vi "GetRemoteVIRef.vi"(8 "ErrorIn":errorcluster, 11 "YActorIn":refnum<class "YActor.lvclass">) -> (0 "ErrorOut":errorcluster, 1 "CreatedVI":refnum<vi>, 3 "YActorOut":refnum<class "YActor.lvclass">)   [LabVIEW 2021, in "YActor.lvclass"]
uses:
  YActor.lvclass
  YActor.lvclass/YActor.ctl
  InlineReferencePool.ctl
  ExeCmd_sync.vi
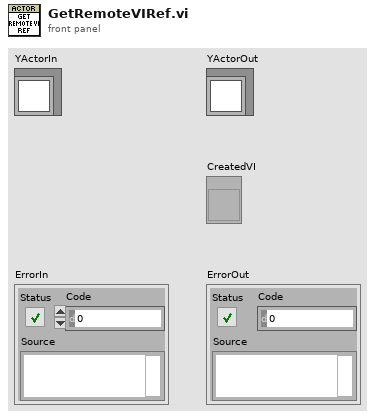
[diagram p1: front panel]
types:
  T1 = typedef "YActor.lvclass/InlineReferencePool.ctl" = enum16{"Add", "ClearAll?"}
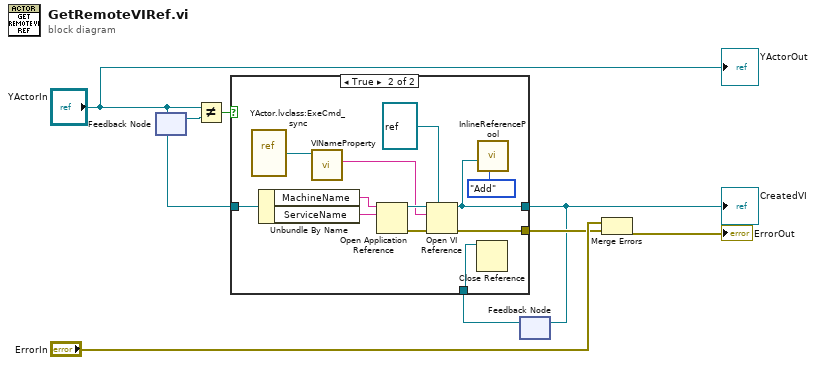
[diagram p0: block diagram]
diagram:
  n1 = feedback #1() -> (w4:refnum<class "YActor.lvclass">)  [unwired: 1 in]
  n2 = feedback-in #1("YActorIn") -> ()
  n3 = Not Equal?(x="YActorIn", y=w4) -> (x != y?=w5:bool)
  n4 = feedback #2() -> (w3:refnum<vi>)  [unwired: 1 in]
  n5 = case shown="True" w5 {
    tunnel: "YActorIn" -> [_ w18]
    tunnel: [w9 w11] -> w2
    tunnel: w3 -> [w9 w10]
    tunnel: [_ w20] -> w6
    frame False {
    }
    frame True {
      n6 = vi-ref "YActor.lvclass:ExeCmd_sync.vi"() -> (w19:refnum<vi>)
      n7 = Unbundle By Name(w18) -> ("MachineName"=w17:string, "ServiceName"=w16:string)
      n8 = call "VINameProperty.vi"("VI in"=w19) -> ("Name"=w14:string)  [unwired: 9 in, 1 out]
      n9 = Open Application Reference(10:w16, 11:w17) -> (0:w21:errorcluster, 3:w15:refnum<vi>)  [unwired: 2 in]
      n10 = Open VI Reference(type specifier VI Refnum (for type only)=refnum<vi> refnum, application reference (local)=w15, vi path=w14, error in (no error)=w21) -> (vi reference=w11:refnum<vi>, error out=w20:errorcluster)  [unwired: 2 in]
      n11 = Close Reference(reference=w10) -> ()  [unwired: 1 in, 1 out]
      n12 = call "InlineReferencePool.vi"("functions"=InlineReferencePool."Add", "inline vi ref"=w11) -> ()  [unwired: 8 in, 2 out]
    }
  }
  "CreatedVI" <- w2
  n13 = feedback-in #2(w2) -> ()
  n14 = Merge Errors("ErrorIn", w6) -> (→"ErrorOut":errorcluster)
  "YActorOut" <- "YActorIn"
